vi "execute_illustrative_command.vi"(2 "input_command":string, 3 "input_machine_reference.lvclass":refnum<class "machine.lvclass">) -> (1 "output_machine_reference.lvclass":refnum<class "machine.lvclass">)   [LabVIEW 2014, in "machine.lvclass"]
uses:
  machine.lvclass
  machine.lvclass/machine.ctl
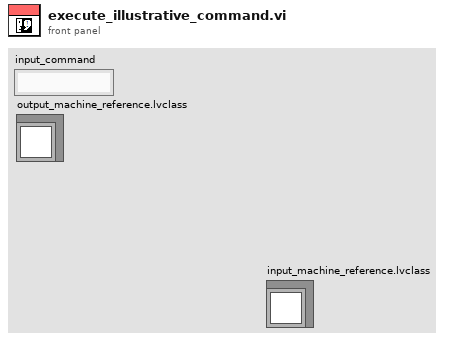
[diagram p1: front panel]
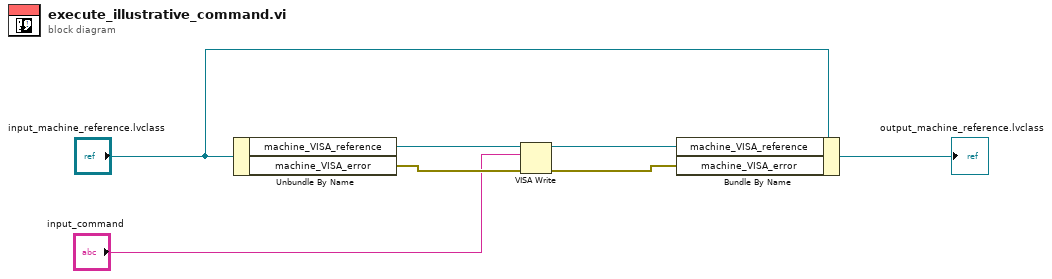
[diagram p0: block diagram]
diagram:
  n1 = Unbundle By Name("input_machine_reference.lvclass") -> ("machine_VISA_reference"=w7:refnum<visa-resource-name>, "machine_VISA_error"=w6:errorcluster)
  n2 = VISA Write(VISA resource name=w7, write buffer="input_command", error in (no error)=w6) -> (VISA resource name out=w3:refnum<visa-resource-name>, error out=w2:errorcluster)  [unwired: 1 out]
  n3 = Bundle By Name(cluster="input_machine_reference.lvclass", "machine_VISA_reference"=w3, "machine_VISA_error"=w2) -> (→"output_machine_reference.lvclass":refnum<class "machine.lvclass">)
